vi "GetScriptNames.vi"(8 "error in":errorcluster, 11 "ConfigINIFiles":path[](array[path])) -> (0 "error out":errorcluster, 3 "Script Names":string[](array[string]))   [LabVIEW 2018]
doc: "This VI retrieves all the section names in the INI file(s)."
uses:
  <vilib>/Utility/config.llb/NI_LVConfig.lvlib
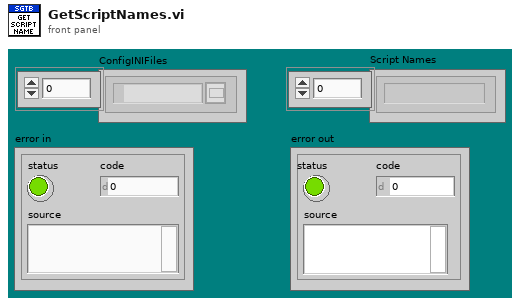
[diagram p1: front panel]
types:
  T1 = typedef "NI_LVConfig.lvlib/Config Data RefNum.ctl" = refnum<k1>
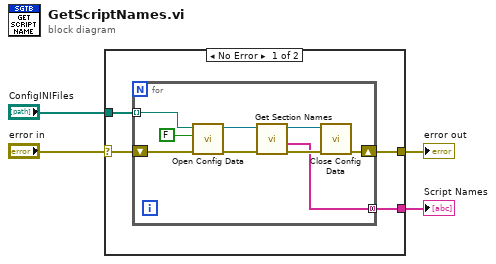
[diagram p0: block diagram]
diagram:
  n1 = case shown="No Error" "error in" {
    selector: "error in" -> [w8 w18]
    tunnel: [w7 w18] -> w1
    tunnel: "ConfigINIFiles" -> [w6 _]
    tunnel: [w5 _] -> w3
    frame No Error {
      n2 = for {
        shift-right: [w16] -> w7
        shift-left: w8 -> [w17]
        tunnel: w6 -> [w14] mode=indexing
        tunnel: [w9] -> w5 mode=concatenating
        n3 = call <vilib>:"Open Config Data.vi"("error in (no error)"=w17, "create file if necessary (T)"=FALSE, "configuration file path"=w14) -> ("error out"=w12:errorcluster, "refnum"=w13:T1)  [unwired: 6 in, 1 out]
        n4 = call <vilib>:"Get Section Names.vi"("error in (no error)"=w12, "refnum"=w13) -> ("error out"=w11:errorcluster, "section names"=w9:string[], "refnum out"=w10:T1)  [unwired: 7 in]
        n5 = call <vilib>:"Close Config Data.vi"("error in (no error)"=w11, "refnum"=w10) -> ("error out"=w16:errorcluster)  [unwired: 8 in, 1 out]
      }
    }
    frame Error {
    }
  }
  "error out" <- w1
  "Script Names" <- w3
